vi "CCC Load Tag List.vi"(8 "error in":errorcluster, 10 "Target Name":string, 11 "TCE Config File Path":path) -> (0 "error out":errorcluster, 3 "CCC Tag List":T1[](array[typedef]))   [LabVIEW 2010]
uses:
  ccc_TagConfiguration.ctl
  <vilib>/NI/Current Value Table/Compatibility/_SubVIs/TypeDefs/cvt_Data Types.ctl
  ccc_TagDirection.ctl
  NI_CCC.lvlib
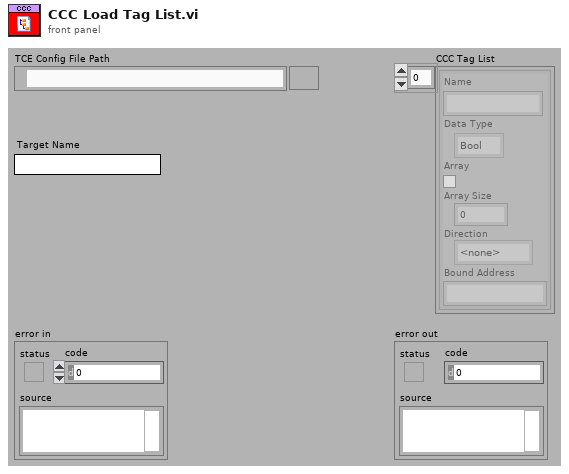
[diagram p1: front panel]
types:
  T1 = typedef "ccc_TagConfiguration.ctl" = cluster{"Name":string, "Data Type":T2, "Array":bool, "Array Size":u32, "Direction":T3, "Bound Address":string}
  T2 = typedef "cvt_Data Types.ctl" = enum16{"Bool", "U8", "I32", "Double", "String", "Enum"}
  T3 = typedef "ccc_TagDirection.ctl" = enum32{"<none>", "Read", "Write"}
  T4 = typedef "NI_CCC.lvlib/Tag Configuration.ctl" = cluster{"name":string, "data type":T5, "direction":T6, "bound address":string}
  T5 = typedef "Current Value Table.lvlib/Data Types.ctl" = enum16{"Double", "Single", "I64", "I32", "I16", "I8", "U64", "U32", "U16", "U8", "String", "Boolean"}
  T6 = typedef "NI_CCC.lvlib/Tag Direction.ctl" = enum32{"<none>", "Read", "Write"}
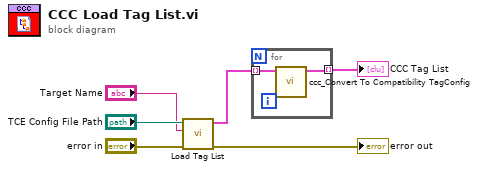
[diagram p0: block diagram]
diagram:
  n1 = call "Load Tag List.vi"("error in"="error in", "target name"="Target Name", "TCE config file path"="TCE Config File Path") -> ("error out"=→"error out":errorcluster, "tag list"=w2:T4[])  [unwired: 7 in]
  n2 = for {
    tunnel: w2 -> [w8] mode=indexing
    tunnel: [w7] -> w1 mode=indexing
    n3 = call "ccc_Convert To Compatibility TagConfig.vi"("new tag"=w8) -> ("old tag"=w7:T1)  [unwired: 10 in]
  }
  "CCC Tag List" <- w1
